vi "開啟圖片(2D).vi"(0 "ImageNameArray":string[](array[string])=["Source"], 5 "影像數量":i32=1, 11 "error In":errorcluster) -> (3 "ImagePath":path[](array[path]), 4 "Image2DArray":T1[][](array[typedef]), 6 "ImageNameNumber":i32, 8 "ImagePathNumber":i32, 10 "ImageOutNameArray":string[](array[string]), 15 "error out":errorcluster)   [LabVIEW 2015]
uses:
  <vilib>/vision/Image Controls.llb/IMAQ Image.ctl
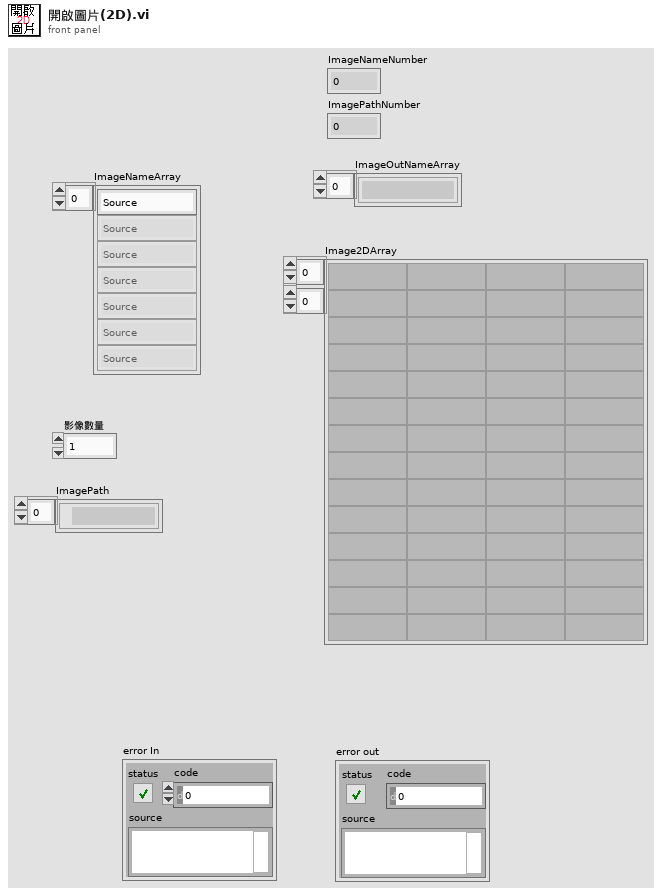
[diagram p1: front panel]
types:
  T1 = typedef "IMAQ Image.ctl" = refnum<image>
  T2 = typedef "Image action.ctl" = enum16{"初始化", "創造記憶體", "寫入圖片", "讀取圖片", "刪除圖片", "等待"}
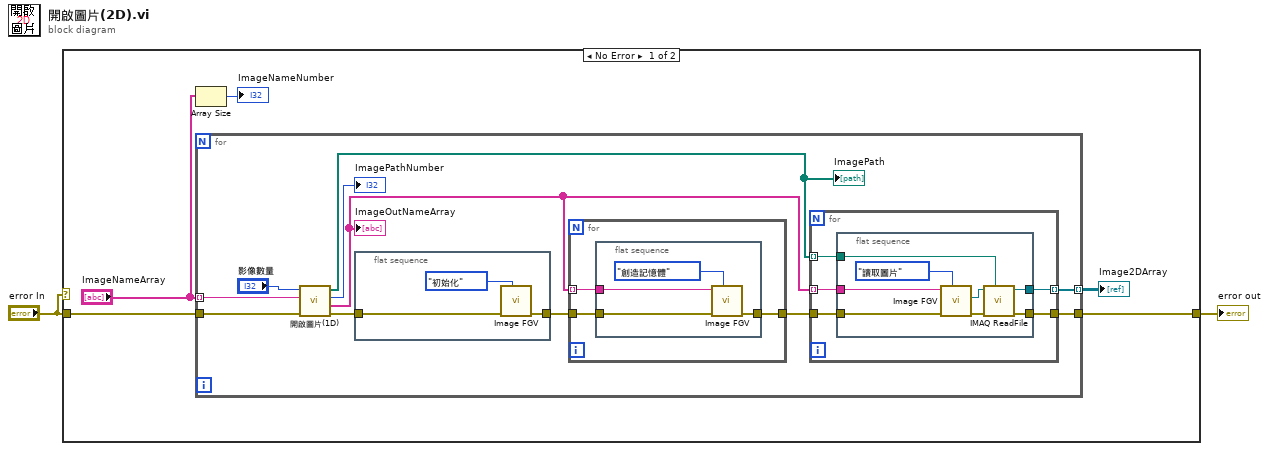
[diagram p0: block diagram]
diagram:
  n1 = case shown="No Error" "error In" {
    tunnel: [w5 w42] -> w2
    tunnel: "error In" -> [w6 w42]
    frame No Error {
      n2 = Array Size(array="ImageNameArray") -> (size(s)=→"ImageNameNumber":i32)
      n3 = for {
        tunnel: "ImageNameArray" -> [w13] mode=indexing
        tunnel: [w12] -> w7 mode=indexing
        tunnel: w6 -> [w10]
        tunnel: [w9] -> w5
        n4 = call "開啟圖片(1D).vi"("error In"=w10, "影像數量"=w13, "Image Name"="影像數量") -> ("error out"=w11:errorcluster, "ImageOutNameArray"=w14:string[], "ImagePathNumber"=→"ImagePathNumber":i32, "ImagePath"=w15:path[])  [unwired: 5 in]
        "ImageOutNameArray" <- w14
        "ImagePath" <- w15
        n5 = flat-sequence {
          tunnel: [w40] -> w18
          tunnel: w11 -> [w39]
          frame #0 {
            n6 = call "Image FGV.vi"("Image action"=Image_action."初始化", "error in (no error)"=w39) -> ("error out"=w40:errorcluster)  [unwired: 8 in, 1 out]
          }
        }
        n7 = for {
          tunnel: w18 -> [w34]
          tunnel: w14 -> [w33] mode=indexing
          tunnel: [w32] -> w16
          n8 = flat-sequence {
            tunnel: w34 -> [w37]
            tunnel: w33 -> [w36]
            tunnel: [w35] -> w32
            frame #0 {
              n9 = call "Image FGV.vi"("Image action"=Image_action."創造記憶體", "error in (no error)"=w37, "圖片名稱"=w36) -> ("error out"=w35:errorcluster)  [unwired: 7 in, 1 out]
            }
          }
        }
        n10 = for {
          tunnel: w16 -> [w23]
          tunnel: w14 -> [w22] mode=indexing
          tunnel: w15 -> [w21] mode=indexing
          tunnel: [w20] -> w12 mode=indexing
          tunnel: [w19] -> w9
          n11 = flat-sequence {
            tunnel: w23 -> [w30]
            tunnel: w22 -> [w29]
            tunnel: w21 -> [w28]
            tunnel: [w26] -> w20
            tunnel: [w24] -> w19
            frame #0 {
              n12 = call "Image FGV.vi"("Image action"=Image_action."讀取圖片", "error in (no error)"=w30, "圖片名稱"=w29) -> ("error out"=w25:errorcluster, "Image Out"=w27:T1)  [unwired: 7 in]
              n13 = call "IMAQ ReadFile"("File Path"=w28, "error in (no error)"=w25, "Image"=w27) -> ("error out"=w24:errorcluster, "Image Out"=w26:T1)  [unwired: 4 in, 3 out]
            }
          }
        }
      }
      "Image2DArray" <- w7
    }
    frame Error {
    }
  }
  "error out" <- w2
